vi "stepNhold.vi"() -> ()   [LabVIEW 2020]
panel:
  in  "Motor control":enum16{"BLM motor", "IMS motor"}(ring)
  in  "stop dataacq":bool
  in  "loop":string="1"
  in  "T0 336":refnum<visa-resource-name>="GPIB0::12::INSTR"
  out "waiting (s)":dbl
  in  "meas time (s)":dbl=10.0
  in  "rate(T/min)":dbl=0.3 min=0.0
  in  "Power supply":enum16{"SCM1 PS", "Resistive PS"}(ring)
  in  "Exp. Mode":u16(ring)=1 items=["T sweep", "H sweep", "Angle sweep", "Other"]
  in  "Pass":bool
  in  "NML Data Acquisition VI":string(combo)="NML Data Acquisition-New.vi"
  out "stable":bool
  out "Reading":dbl=-999.99 format="%#_4g"
  out "done":i32
  in  "Finish":bool
  out "On Target":bool=TRUE
  in  "Target error":dbl=0.002 format="%#_13g"
  in  "timeout (s)":dbl=600.0
  out "time passed (s)":dbl format="%#_4g"
  out "status":string="Temp reached. Wait for stability"
  out "completed":bool
  out "table":dbl[][](array[numeric])=[[0.01, 0.41], [0.05, 0.32], [0.1, 0.33], [6.0, 2.0], [8.0, 2.0], [10.0, 2.0], [14.0, 2.0], [15.0, 2.0], [16.0, 2.0], [17.0, 2.0], [18.0, 2.0], [19.0, 2.0], [20.0, 2.0], [21.0, 2.0], [25.0, 1.0], [26.0, 2.0], [28.0, 2.0], [30.0, 2.0], [28.0, 2.0], [26.0, 2.0], [25.0, 2.0], [21.0, 1.0], [20.0, 2.0], [19.0, 2.0], [18.0, 2.0], [17.0, 2.0], [16.0, 2.0], [15.0, 2.0], [14.0, 2.0], [11.0, 1.0], [10.0, 2.0], [8.0, 2.0], [6.0, 2.0], [4.0, 2.0], [2.0, 2.0], [0.0, 2.0]]
  in  "Set T, wait (m)":string="0.01 0.41\n0.05 0.32\n0.1 0.33\n6 2\n8 2\n10 2\n14 2\n15 2\n16 2\n17 2\n18 2\n19 2\n20 2\n21 2\n25 1\n26 2\n28 2\n30 2\n28 2\n26 2\n25 2\n21 1\n20 2\n19 2\n18 2\n17 2\n16 2\n15 2\n14 2\n11 1\n10 2\n8 2\n6 2\n4 2\n2 2\n0 2" caption="Set Field(T), rate(T/min) (defualt rate: first row value)"
  in  "Use\nTable":bool
  in  "stable wait":dbl=10.0
  out "Target value":dbl=-1000.0
  in  "step":dbl=0.05
  in  "Final Target":dbl=1.0
  in  "Initial Target":dbl
  # "Step and Hold temperature, field or angle.\nData will be collected only when 'hold' state.\n\nField and Angle: There is no stability check\nTemp: Tcheck.vi check the stability.\n\nTiming\nstable wait: waiting time after 'hold' condition is met.\nmeas time (s): duration for data collection.\ntimeout (s): max time allowed to reach 'hold' condition."
  # "(s)"
  # "If ON, when the final target is reached,\ndata acq will be stopped\nand the data will be saved\n\nOtherwise, it will be paused."
  # "Txb: T's (0, hot, col) with heater off\nTxh: T's with heater on"
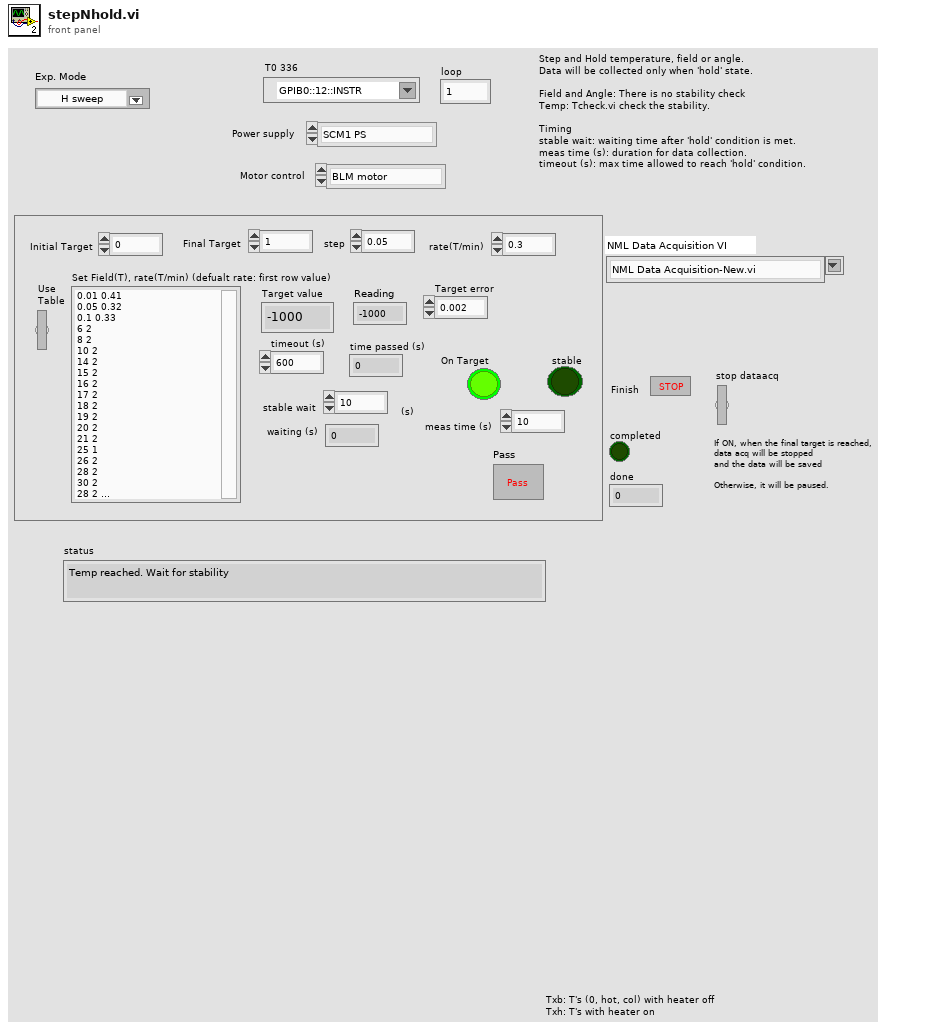
[diagram p1: front panel]
types:
  T1 = enum32{"New", "Stop", "Trigger", "Delta Trigger", "Run", "Pause"}
  T2 = enum32{"New", "Stop", "Trigger", "Delta Trigger", "Run", "Pause", "comments", "Started?"}
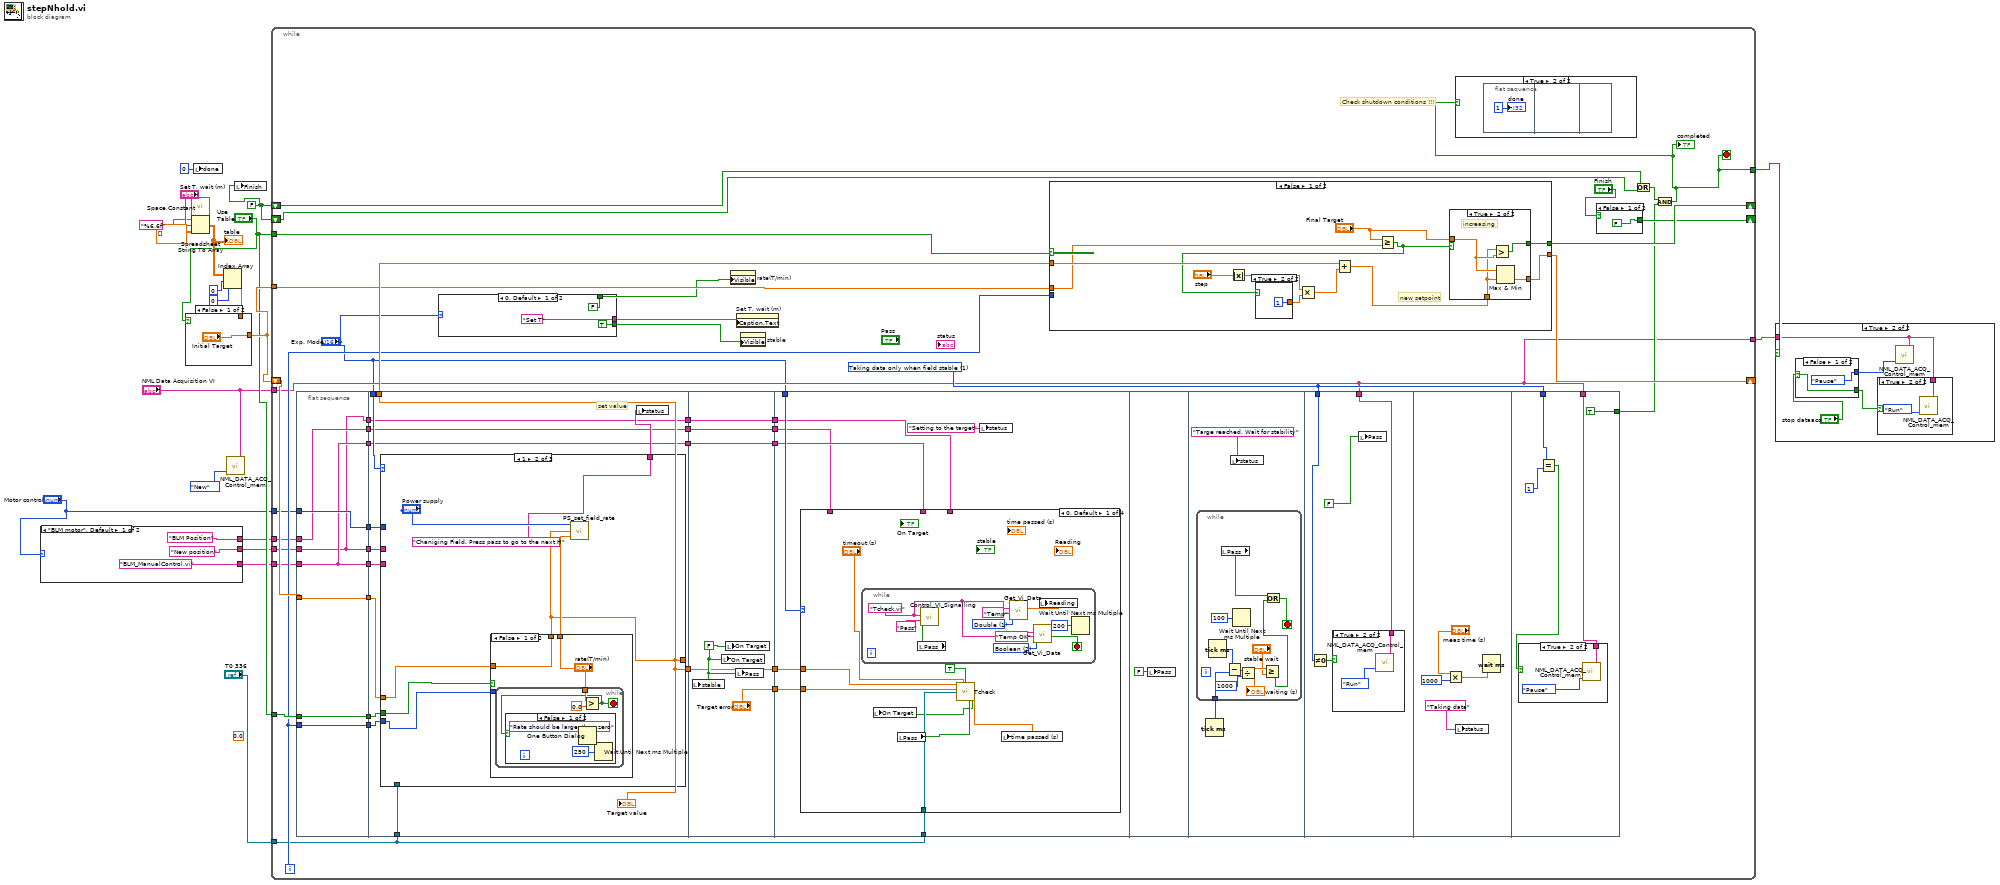
[diagram p0: block diagram]
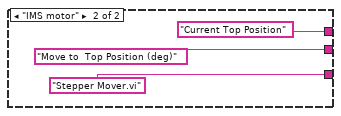
[diagram p2: hidden frame]
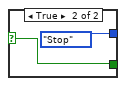
[diagram p5: hidden frame]
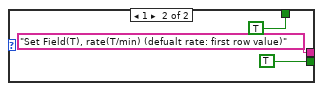
[diagram p7: hidden frame]
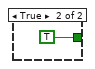
[diagram p9: hidden frame]
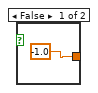
[diagram p10: hidden frame]
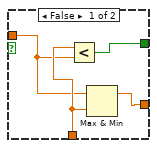
[diagram p11: hidden frame]
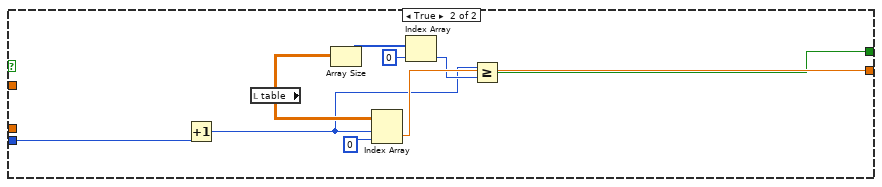
[diagram p12: hidden frame]
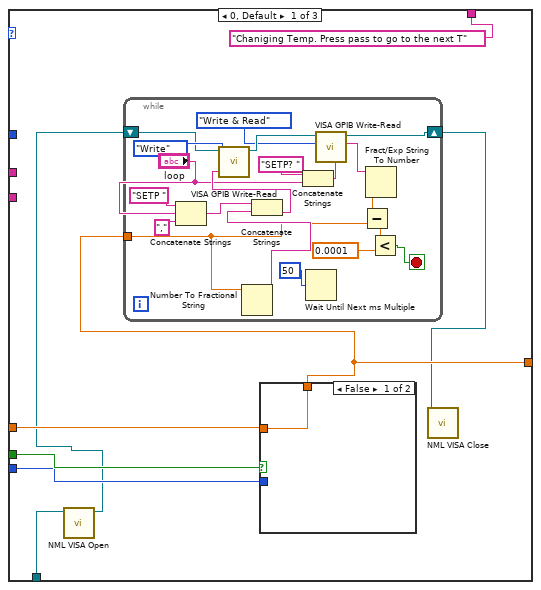
[diagram p13: hidden frame]
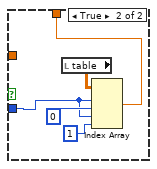
[diagram p14: hidden frame]
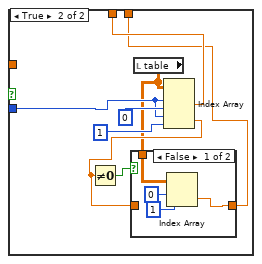
[diagram p16: hidden frame]
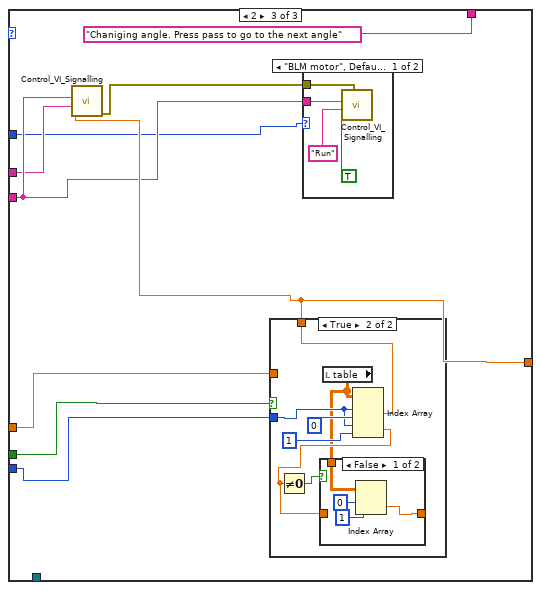
[diagram p18: hidden frame]
diagram:
  (unwired) 0.0 ("setT")
  w11 = FALSE
  n1 = case shown="\"BLM motor\", Default" "Motor control" {
    tunnel: ["BLM_ManualControl.vi" ("Target VI name") "Stepper Mover.vi" ("Target VI name")] -> w5
    tunnel: ["New position" ("Control Name") "Move to  Top Position (deg)" ("Control Name")] -> w4
    tunnel: ["BLM Position" "Current Top Position"] -> w2
    frame "BLM motor", Default {
    }
    frame "IMS motor" {
    }
  }
  n2 = call <vilib>:"Space Constant.vi"() -> ("String"=w17:string)
  n3 = Spreadsheet String To Array(delimiter (Tab)=w17, format string="%6.6f", spreadsheet string="Set T, wait (m)", array type (2D Dbl)=dbl[][] []) -> (array=w16:dbl[][])
  "table" <- w16
  n4 = local write "done"(0 ("done")) -> ()
  n5 = Index Array(array=w16, index (row)=0, index (col)=0 ("disabled index (col)")) -> (element=w13:dbl)
  n6 = case shown="False" "Use\nTable" {
    tunnel: ["Initial Target" w29] -> w21
    tunnel: w13 -> [_ w29]
    frame False {
    }
    frame True {
    }
  }
  n7 = call "NML_DATA_ACQ_Control_mem.vi"("NML Data Acquisition VI"="NML Data Acquisition VI", "Enum"=T1."New") -> ()  [unwired: 3 in, 1 out]
  n8 = local write "Finish"(w11) -> ()
  n9 = while {
    shift-right: [w71] -> _
    shift-left: w21 -> [w73]
    tunnel: w21 -> [w70]
    tunnel: "Use\nTable" -> [w69]
    tunnel: "Use\nTable" -> [w68]
    shift-right: [w66] -> _
    shift-left: w11 -> [w62]
    shift-right: [w63] -> _
    shift-left: w11 -> [w61]
    tunnel: "NML Data Acquisition VI" -> [w50]
    tunnel: [w51] -> w7
    tunnel: [w50] -> w6
    tunnel: w5 -> [w46]
    tunnel: w4 -> [w45]
    tunnel: "Motor control" -> [w42]
    tunnel: w2 -> [w38]
    tunnel: "T0 336" -> [w30]
    i -> [w67]
    stop <- w51 stop-if-true
    w65 = u16 1 items=["No interrupt", "Taking data only when field stable", "Taking data always"] ("Data acqusition ? (Run and Pause)")
    # "Check shutdown conditions !!!"
    n10 = flat-sequence {
      tunnel: w67 -> [w117]
      tunnel: w68 -> [w118]
      tunnel: w73 -> [w119]
      tunnel: [w119] -> w54
      tunnel: [w118] -> w53
      tunnel: [w117] -> w52
      tunnel: [w115] -> w47
      tunnel: w46 -> [w115]
      tunnel: w45 -> [w113]
      tunnel: [w113] -> w44
      tunnel: [w116] -> w43
      tunnel: w42 -> [w116]
      tunnel: [w115] -> w39
      tunnel: w38 -> [w114]
      tunnel: [w114] -> w37
      tunnel: [w113] -> w32
      tunnel: [w126] -> w72
      tunnel: "Exp. Mode" -> [w128]
      tunnel: w54 -> [w130]
      tunnel: w53 -> [w132]
      tunnel: w52 -> [w131]
      tunnel: w30 -> [w127]
      tunnel: [w126] -> w49
      tunnel: w47 -> [w125]
      tunnel: w44 -> [w124]
      tunnel: w43 -> [w123]
      tunnel: [w122] -> w40
      tunnel: w39 -> [w122]
      tunnel: w37 -> [w121]
      tunnel: [w121] -> w36
      tunnel: [w120] -> w33
      tunnel: w32 -> [w120]
      tunnel: ["Target error"] -> w60
      tunnel: w49 -> [w223]
      tunnel: [w223] -> w48
      tunnel: [w222] -> w41
      tunnel: w40 -> [w222]
      tunnel: w36 -> [w221]
      tunnel: [w221] -> w35
      tunnel: [w220] -> w34
      tunnel: w33 -> [w220]
      tunnel: "Exp. Mode" -> [w233]
      tunnel: w60 -> [w232]
      tunnel: w48 -> [w230]
      tunnel: w41 -> [w229]
      tunnel: w35 -> [w228]
      tunnel: w34 -> [w227]
      tunnel: w30 -> [w226]
      tunnel: w65 -> [w311]
      tunnel: w50 -> [w310]
      tunnel: w65 -> [w324]
      tunnel: [TRUE] -> w55
      tunnel: w50 -> [w320]
      frame #0 {
      }
      frame #1 {
        # "set value"
        n11 = case shown="1" w128 {
          tunnel: w132 -> [w140 w170 w201]
          tunnel: w131 -> [w139 w173 w202]
          tunnel: w130 -> [w138 w169 w200]
          tunnel: [w137 w168 w198] -> w126
          tunnel: ["Chaniging Temp. Press pass to go to the next T" ("status") "Chaniging Field. Press pass to go to the next H" ("status") "Chaniging angle. Press pass to go to the next angle" ("status")] -> w129
          tunnel: w127 -> [w135 _ _]
          tunnel: w125 -> [_ _ w196]
          tunnel: w124 -> [_ _ w195]
          tunnel: w123 -> [_ _ w194]
          frame 0, Default {
            n12 = call "NML VISA Open.vi"("VISA resource name"=w135) -> ("VISA resource name out"=w134:refnum<visa-resource-name>)  [unwired: 9 in, 1 out]
            n13 = case shown="False" w140 {
              tunnel: [w161 w165] -> w137
              tunnel: w139 -> [_ w163]
              tunnel: w138 -> [w161 _]
              frame False {
              }
              frame True {
                n14 = local read "table"() -> (w166:dbl[][])
                n15 = Index Array(array=w166, index (row) #1=w163, index (col) #1=0 ("disabled index (row)"), index (row) #2=w163, index (col) #2=1 ("disabled index (col)")) -> (element #1=w165:dbl)  [unwired: 1 out]
              }
            }
            n16 = while {
              tunnel: w137 -> [w149]
              shift-right: [w141] -> w133
              shift-left: w134 -> [w157]
              stop <- w148 stop-if-true
              n17 = Concatenate Strings("SETP " ("Command"), "loop", "," ("Command")) -> (w145:string)
              n18 = Number To Fractional String(number=w149) -> (F-format string=w159:string)  [unwired: 3 in]
              n19 = Concatenate Strings(w145, w159) -> (w158:string)
              n20 = call "VISA GPIB Write-Read.vi"("Command"=w158, "Action"=enum16{"Write", "Read", "Write & Read"}."Write", "VISA resource name"=w157) -> ("dup VISA Session"=w156:refnum<visa-resource-name>)  [unwired: 5 in, 3 out]
              n21 = Concatenate Strings("SETP? " ("Command"), "loop") -> (w143:string)
              n22 = Wait Until Next ms Multiple(millisecond multiple=u32 50) -> ()  [unwired: 1 out]
              n23 = call "VISA GPIB Write-Read.vi"("Command"=w143, "Action"=enum16{"Write", "Read", "Write & Read"}."Write & Read", "VISA resource name"=w156) -> ("String Returned"=w154:string, "dup VISA Session"=w141:refnum<visa-resource-name>)  [unwired: 5 in, 2 out]
              n24 = Fract/Exp String To Number(string=w154) -> (number=w153:dbl)  [unwired: 3 in, 1 out]
              n25 = Subtract(x=w153, y=w149) -> (x-y=w152:dbl)
              n26 = Less?(x=w152, y=0.0001) -> (x < y?=w148:bool)
            }
            n27 = call "NML VISA Close.vi"("VISA resource name"=w133) -> ()  [unwired: 10 in, 1 out]
          }
          frame 1 {
            n28 = case shown="False" w170 {
              tunnel: ["rate(T/min)" w182] -> w171
              tunnel: w173 -> [_ w187]
              tunnel: [w175 w185] -> w168
              tunnel: w169 -> [w175 _]
              frame False {
                n29 = while {
                  tunnel: "rate(T/min)" -> [w178]
                  stop <- w176 stop-if-true
                  n30 = Greater?(x=w178, y=0.0) -> (0:w176:bool)
                  n31 = case shown="False" w176 {
                    frame False {
                      n32 = One Button Dialog(message="Rate should be larger than zero") -> ()  [unwired: 1 in, 1 out]
                      n33 = Wait Until Next ms Multiple(millisecond multiple=u32 250) -> ()  [unwired: 1 out]
                    }
                    frame True {
                    }
                  }
                }
              }
              frame True {
                n34 = local read "table"() -> (w181:dbl[][])
                n35 = Index Array(array=w181, index (row) #1=w187, index (col) #1=0 ("disabled index (row)"), index (row) #2=w187, index (col) #2=1 ("disabled index (col)")) -> (element #1=w185:dbl, element #2=w183:dbl)
                n36 = Not Equal To 0?(x=w183) -> (x != 0?=w184:bool)
                n37 = case shown="False" w184 {
                  tunnel: [w189 w193] -> w182
                  tunnel: w183 -> [_ w193]
                  tunnel: w181 -> [w192 _]
                  frame False {
                    n38 = Index Array(array=w192, index (row)=0, index (col)=1 ("disabled index (col)")) -> (element=w189:dbl)
                  }
                  frame True {
                  }
                }
              }
            }
            n39 = call "PS_set_field_rate.vi"("ramping rate"=w171, "set point"=w168, "Power supply"="Power supply") -> ()
          }
          frame 2 {
            n40 = case shown="True" w201 {
              tunnel: w202 -> [_ w213]
              tunnel: [w207 w211] -> w198
              tunnel: w200 -> [w207 _]
              frame False {
              }
              frame True {
                n41 = local read "table"() -> (w208:dbl[][])
                n42 = Index Array(array=w208, index (row) #1=w213, index (col) #1=0 ("disabled index (row)"), index (row) #2=w213, index (col) #2=1 ("disabled index (col)")) -> (element #1=w211:dbl, element #2=w209:dbl)
                n43 = Not Equal To 0?(x=w209) -> (x != 0?=w210:bool)
                n44 = case shown="False" w210 {
                  tunnel: [w215 w219] -> _
                  tunnel: w209 -> [_ w219]
                  tunnel: w208 -> [w218 _]
                  frame False {
                    n45 = Index Array(array=w218, index (row)=0, index (col)=1 ("disabled index (col)")) -> (element=w215:dbl)
                  }
                  frame True {
                  }
                }
              }
            }
            n46 = call "Control_VI_Signalling.vi"("Input Value"=w198, "Control Name"=w195, "Target VI name"=w196) -> ("error out"=w197:errorcluster)  [unwired: 8 in]
            n47 = case shown="\"BLM motor\", Default" w194 {
              tunnel: w197 -> [w204 _]
              tunnel: w196 -> [w203 _]
              frame "BLM motor", Default {
                n48 = call "Control_VI_Signalling.vi"("error in (no error)"=w204, "Input Value"=TRUE ("Use\nTable"), "Control Name"="Run", "Target VI name"=w203) -> ()  [unwired: 7 in, 1 out]
              }
              frame "IMS motor" {
              }
            }
          }
        }
        "Target value" <- w126
        n49 = local write "status"(w129) -> ()
      }
      frame #2 {
        w224 = FALSE ("Pass")
        n50 = local write "stable"(w224) -> ()
        n51 = local write "On Target"(w224) -> ()
        n52 = local write "On Target"(w224) -> ()
        n53 = local write "Pass"(w224) -> ()
      }
      frame #3 {
        n54 = case shown="0, Default" w233 {
          tunnel: w230 -> [w241 _ _ _]
          tunnel: w232 -> [w240 w253 w277 _]
          tunnel: w226 -> [w239 _ _ _]
          tunnel: w229 -> [_ _ w275 _]
          tunnel: w228 -> [_ _ w274 _]
          tunnel: w227 -> [_ _ w273 _]
          frame 0, Default {
            n55 = while {
              stop <- w242 stop-if-true
              w249 = u16 2 items=["String", "Double", "Boolean", "Variant"] ("Data Type")
              w250 = u16 1 items=["String", "Double", "Boolean", "Variant"] ("Data Type")
              w246 = "Tcheck.vi" ("Target VI name")
              n56 = local read "Pass"() -> (w251:bool)
              n57 = call "Control_VI_Signalling.vi"("Input Value"=w251, "Control Name"="Pass", "Target VI name"=w246) -> ()  [unwired: 8 in, 1 out]
              n58 = call "Get_Vi_Data.vi"("Data Type"=w250, "VI name"=w246, "Control Name"="Temp" ("VI name")) -> ("Data (Double)"=w243:dbl)  [unwired: 4 in, 4 out]
              n59 = call "Get_Vi_Data.vi"("Data Type"=w249, "VI name"=w246, "Control Name"="Temp OK" ("VI name")) -> ("Boolean"=w242:bool)  [unwired: 4 in, 4 out]
              n60 = local write "Reading"(w243) -> ()
              n61 = Wait Until Next ms Multiple(millisecond multiple=u32 200) -> ()  [unwired: 1 out]
            }
            n62 = local read "Pass"() -> (w237:bool)
            n63 = call "Tcheck.vi"("TargetT"=w241, "timeout (s)"="timeout (s)", "Direct reading"=TRUE, "target T\nDT error"=w240, "VISA resource name"=w239, "Pass"=w237) -> ("Temp close to\nTarget T"=w235:bool, "Temp"=w236:dbl)  [unwired: 6 in, 2 out]
            n64 = local write "On Target"(w235) -> ()
            n65 = local write "time passed (s)"(w236) -> ()
          }
          frame 1 {
            n66 = Tick Count (ms)() -> (millisecond timer value=w252:u32)
            n67 = while {
              tunnel: w253 -> [w261]
              tunnel: w252 -> [w258]
              tunnel: [w254] -> _
              stop <- w254 stop-if-true
              w266 = u16 1 items=["String", "Double", "Boolean", "Variant"] ("Data Type")
              w269 = "PS Control.vi" ("VI name")
              n68 = Wait Until Next ms Multiple(millisecond multiple=u32 200 ("200")) -> ()  [unwired: 1 out]
              n69 = Tick Count (ms)() -> (millisecond timer value=w259:u32)
              n70 = call "Get_Vi_Data.vi"("Data Type"=w266, "VI name"=w269, "Control Name"="Field [T]") -> ("error out"=w268:errorcluster, "Data (Double)"=w260:dbl)  [unwired: 4 in, 3 out]
              n71 = Subtract(x=w259, y=w258) -> (x-y=w257:u32)
              n72 = local write "Reading"(w260) -> ()
              n73 = call "Get_Vi_Data.vi"("error in (no error) 2"=w268, "Data Type"=w266, "VI name"=w269, "Control Name"="Setpoint [T]") -> ("Data (Double)"=w265:dbl)  [unwired: 3 in, 4 out]
              n74 = Divide(x=w257, y=u32 1000) -> (x/y=w255:dbl)
              n75 = Subtract(x=w265, y=w260) -> (x-y=w263:dbl)
              n76 = Absolute Value(x=w263) -> (abs(x)=w264:dbl)
              n77 = local write "time passed (s)"(w255) -> ()
              n78 = local read "Pass"() -> (w272:bool)
              n79 = Less?(x=w264, y=w261) -> (x < y?=w262:bool)
              n80 = Or(x=w262, y=w272) -> (x .or. y?=w254:bool)
              n81 = local write "On Target"(w254) -> ()
            }
          }
          frame 2 {
            n82 = Tick Count (ms)() -> (millisecond timer value=w276:u32)
            n83 = while {
              tunnel: w277 -> [_]
              tunnel: w276 -> [w285]
              tunnel: w275 -> [w280]
              tunnel: w274 -> [w279]
              tunnel: w273 -> [w278]
              stop <- w288 stop-if-true
              w293 = u16 1 items=["String", "Double", "Boolean", "Variant"] ("Data Type")
              n84 = Wait Until Next ms Multiple(millisecond multiple=u32 200 ("200")) -> ()  [unwired: 1 out]
              n85 = Tick Count (ms)() -> (millisecond timer value=w286:u32)
              n86 = call "Get_Vi_Data.vi"("Data Type"=w293, "VI name"=w280, "Control Name"=w279) -> ("error out"=w294:errorcluster, "Data (Double)"=w287:dbl)  [unwired: 4 in, 3 out]
              n87 = Subtract(x=w286, y=w285) -> (x-y=w284:u32)
              n88 = local write "Reading"(w287) -> ()
              n89 = call "Get_Vi_Data.vi"("error in (no error) 2"=w294, "Data Type"=w293, "VI name"=w280, "Control Name"=w278) -> ("Data (Double)"=w292:dbl)  [unwired: 3 in, 4 out]
              n90 = Divide(x=w284, y=u32 1000) -> (x/y=w282:dbl)
              n91 = Subtract(x=w292, y=w287) -> (x-y=w290:dbl)
              n92 = Absolute Value(x=w290) -> (abs(x)=w291:dbl)
              n93 = local write "time passed (s)"(w282) -> ()
              n94 = local read "Pass"() -> (w296:bool)
              n95 = Less?(x=w291, y=2.0) -> (x < y?=w289:bool)
              n96 = Or(x=w289, y=w296) -> (x .or. y?=w288:bool)
              n97 = local write "On Target"(w288) -> ()
            }
          }
          frame 3 {
          }
        }
        n98 = local write "status"("Setting to the target" ("status")) -> ()
      }
      frame #4 {
        n99 = local write "Pass"(FALSE ("Pass")) -> ()
      }
      frame #5 {
        n100 = Tick Count (ms)() -> (millisecond timer value=w298:u32)
        n101 = while {
          tunnel: w298 -> [w306]
          stop <- w300 stop-if-true
          n102 = Tick Count (ms)() -> (millisecond timer value=w307:u32)
          n103 = local read "Pass"() -> (w301:bool)
          n104 = Subtract(x=w307, y=w306) -> (x-y=w309:u32)
          n105 = Wait Until Next ms Multiple(millisecond multiple=u32 100) -> ()  [unwired: 1 out]
          n106 = Divide(x=w309, y=u32 1000) -> (x/y=w305:dbl)
          "waiting (s)" <- w305
          n107 = Greater Or Equal?(x=w305, y="stable wait") -> (x >= y?=w302:bool)
          n108 = Or(x=w301, y=w302) -> (x .or. y?=w300:bool)
        }
        n109 = local write "status"("Targe reached. Wait for stability" ("status")) -> ()
      }
      frame #6 {
        n110 = Not Equal To 0?(x=w311) -> (x != 0?=w312:bool)
        n111 = case shown="True" w312 {
          tunnel: w310 -> [_ w314]
          frame False {
          }
          frame True {
            n112 = call "NML_DATA_ACQ_Control_mem.vi"("NML Data Acquisition VI"=w314, "Enum"=T1."Run") -> ()  [unwired: 3 in, 1 out]
          }
        }
        n113 = local write "Pass"(FALSE ("Pass")) -> ()
      }
      frame #7 {
        n114 = Multiply(x="meas time (s)", y=u32 1000) -> (x*y=w318:dbl)
        n115 = local write "status"("Taking data" ("status")) -> ()
        n116 = Wait (ms)(milliseconds to wait=w318) -> ()  [unwired: 1 out]
      }
      frame #8 {
        n117 = Equal?(x=w324, y=u16 1) -> (x = y?=w322:bool)
        n118 = case shown="True" w322 {
          tunnel: w320 -> [_ w325]
          frame False {
          }
          frame True {
            n119 = call "NML_DATA_ACQ_Control_mem.vi"("NML Data Acquisition VI"=w325, "Enum"=T2."Pause") -> ()  [unwired: 3 in, 1 out]
          }
        }
      }
    }
    n120 = case shown="0, Default" "Exp. Mode" {
      tunnel: ["Set T" ("Caption.Text") "Set Field(T), rate(T/min) (defualt rate: first row value)" ("Caption.Text")] -> w59
      tunnel: [TRUE ("Visible") TRUE ("Visible")] -> w58
      tunnel: [FALSE ("Visible") TRUE ("Visible")] -> w57
      frame 0, Default {
      }
      frame 1 {
      }
    }
    n121 = property on="rate(T/min)" class="DigNum (strict)"("Visible"=w57) -> ()  [unwired: 2 in, 2 out]
    n122 = property on="Set T, wait (m)" class="Str"("Caption.Text"=w59) -> ()  [unwired: 2 in, 2 out]
    n123 = property on="stable" class="Bool (strict)"("Visible"=w58) -> ()  [unwired: 2 in, 2 out]
    n124 = case shown="False" w69 {
      tunnel: w72 -> [w93 _]
      tunnel: [w92 w107] -> w66
      tunnel: [w90 w112] -> w71
      tunnel: w70 -> [w88 _]
      tunnel: w67 -> [_ w105]
      frame False {
        # "new setpoint"
        n125 = Absolute Value(x="step") -> (abs(x)=w86:dbl)
        n126 = Greater Or Equal?(x="Final Target", y=w88) -> (x >= y?=w84:bool)
        n127 = case shown="True" w84 {
          tunnel: [-1.0 ("x*y") u32 1 ("y")] -> w83
          frame False {
          }
          frame True {
          }
        }
        n128 = Multiply(x=w86, y=w83) -> (x*y=w85:dbl)
        n129 = Add(x=w93, y=w85) -> (x+y=w91:dbl)
        n130 = case shown="True" w84 {
          tunnel: w91 -> [w98 w101]
          tunnel: "Final Target" -> [w97 w102]
          tunnel: [w99 w103] -> w92
          tunnel: [w96 w100] -> w90
          frame False {
            n131 = Less?(x=w98, y=w97) -> (x < y?=w99:bool)
            n132 = Max & Min(x=w97, y=w98) -> (max(x,y)=w96:dbl)  [unwired: 1 out]
          }
          frame True {
            # "increasing"
            n133 = Greater?(x=w101, y=w102) -> (0:w103:bool)
            n134 = Max & Min(x=w102, y=w101) -> (min(x,y)=w100:dbl)  [unwired: 1 out]
          }
        }
      }
      frame True {
        n135 = Increment(x=w105) -> (x+1=w104:i32)
        n136 = local read "table"() -> (w111:dbl[][])
        n137 = Array Size(array=w111) -> (size(s)=w110:i32[])
        n138 = Index Array(array=w111, index (row)=w104, index (col)=0 ("disabled index (col)")) -> (element=w112:dbl)
        n139 = Index Array(array=w110, index=0) -> (element=w108:i32)
        n140 = Greater Or Equal?(x=w104, y=w108) -> (x >= y?=w107:bool)
      }
    }
    n141 = case shown="False" "Finish" {
      tunnel: [FALSE TRUE] -> w63
      frame False {
      }
      frame True {
      }
    }
    n142 = Or(x=w62, y=w61) -> (x .or. y?=w56:bool)
    n143 = And(x=w56, y=w55) -> (x .and. y?=w51:bool)
    "completed" <- w51
    n144 = case shown="True" w51 {
      frame False {
      }
      frame True {
        n145 = flat-sequence {
          frame #0 {
            "done" <- 1 ("done")
          }
          frame #1 {
          }
          frame #2 {
          }
        }
      }
    }
  }
  n146 = case shown="True" w7 {
    tunnel: w6 -> [_ w327]
    frame False {
    }
    frame True {
      n147 = case shown="False" "stop dataacq" {
        selector: "stop dataacq" -> [w333 w335]
        tunnel: [T2."Pause" ("Enum") T2."Stop" ("Enum")] -> w330
        tunnel: [w333 w335] -> w328
        frame False {
        }
        frame True {
        }
      }
      n148 = case shown="True" w328 {
        tunnel: w327 -> [_ w332]
        frame False {
        }
        frame True {
          n149 = call "NML_DATA_ACQ_Control_mem.vi"("NML Data Acquisition VI"=w332, "Enum"=T2."Run") -> ()  [unwired: 3 in, 1 out]
        }
      }
      n150 = call "NML_DATA_ACQ_Control_mem.vi"("NML Data Acquisition VI"=w327, "Enum"=w330) -> ()  [unwired: 3 in, 1 out]
    }
  }
